vi "TEST VI.vi"() -> ()   [LabVIEW 2010]
uses:
  <vilib>/Utility/miscctls.llb/LVRectTypeDef.ctl
  Visualizer.lvlib
panel:
  in  "OK Button 3":bool
  out "File Data 2":waveform(dbl)[](graph)
  in  "OK Button 2":bool
  out "error out":errorcluster
  in  "OK Button":bool
  out "File Data":waveform(dbl)[](graph)
  in  "File Path":path=path "Q:/VIs/Visualizer/sample.wav"
  in  "Number of Samples/ch":i32=-1
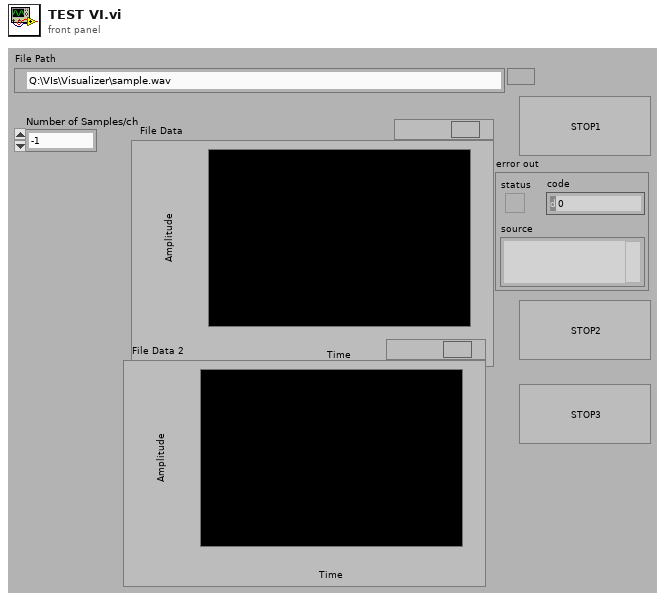
[diagram p1: front panel]
types:
  T1 = typedef "LVRectTypeDef.ctl" = cluster{"Left":i16, "Top":i16, "Right":i16, "Bottom":i16}
  T2 = typedef "Visualizer.lvlib/Visualizer Type ID.ctl" = u32
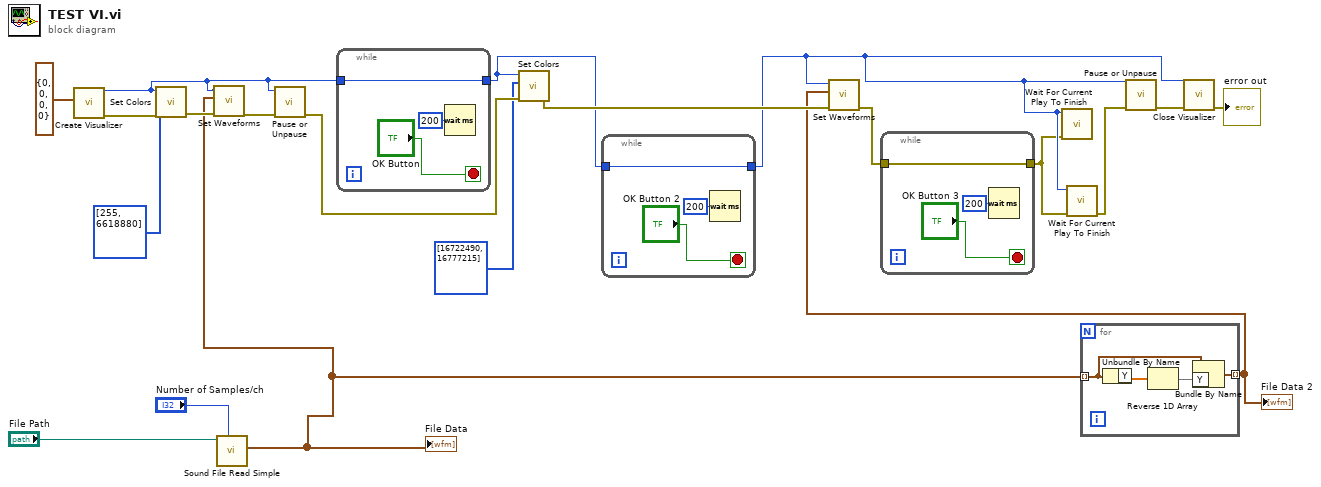
[diagram p0: block diagram]
diagram:
  n1 = call "Create Visualizer.vi"("Front Panel Bounds"=T1 {"Left"=0, "Top"=0, "Right"=0, "Bottom"=0} ("Front Panel Window Bounds")) -> ("error out"=w20:errorcluster, "Visualizer ID"=w14:T2)  [unwired: 9 in]
  n2 = call "Set Colors.vi"("error in (no error)"=w20, "Colors"=u32[] [255, 6618880], "Visualizer ID"=w14) -> ("error out"=w17:errorcluster)  [unwired: 8 in]
  n3 = call <vilib>:"Sound File Read Simple.vi"("number of samples/ch (-1: all)"="Number of Samples/ch", "path"="File Path") -> ("data"=w8:waveform(dbl)[])  [unwired: 6 in, 3 out]
  "File Data" <- w8
  n4 = call "Set Waveforms.vi"("error in (no error)"=w17, "Waveforms"=w8, "Visualizer ID"=w14) -> ("error out"=w15:errorcluster)  [unwired: 8 in]
  n5 = call "Pause or Unpause.vi"("error in (no error)"=w15, "Visualizer ID"=w14) -> ("error out"=w11:errorcluster)  [unwired: 9 in]
  n6 = while {
    tunnel: [w22] -> w6
    tunnel: w14 -> [w22]
    stop <- "OK Button" stop-if-true
    n7 = Wait (ms)(milliseconds to wait=u32 200) -> ()  [unwired: 1 out]
  }
  n8 = call "Set Colors.vi"("error in (no error)"=w11, "Colors"=u32[] [16722490, 16777215], "Visualizer ID"=w6) -> ("error out"=w7:errorcluster)  [unwired: 8 in]
  n9 = while {
    tunnel: [w25] -> w3
    tunnel: w6 -> [w25]
    stop <- "OK Button 2" stop-if-true
    n10 = Wait (ms)(milliseconds to wait=u32 200) -> ()  [unwired: 1 out]
  }
  n11 = for {
    tunnel: w8 -> [w29] mode=indexing
    tunnel: [w27] -> w5 mode=indexing
    n12 = Unbundle By Name(w29) -> ("Y"=w30:dbl[])
    n13 = Reverse 1D Array(array=w30) -> (reversed array=w28:dbl[])
    n14 = Bundle By Name(cluster=w29, "Y"=w28) -> (w27:waveform(dbl))
  }
  "File Data 2" <- w5
  n15 = call "Set Waveforms.vi"("error in (no error)"=w7, "Waveforms"=w5, "Visualizer ID"=w3) -> ("error out"=w4:errorcluster)  [unwired: 8 in]
  n16 = while {
    tunnel: [w32] -> w1
    tunnel: w4 -> [w32]
    stop <- "OK Button 3" stop-if-true
    n17 = Wait (ms)(milliseconds to wait=u32 200) -> ()  [unwired: 1 out]
  }
  n18 = call "Wait For Current Play To Finish.vi"("error in (no error)"=w1, "Visualizer ID"=w3) -> ()  [unwired: 8 in, 2 out]
  n19 = call "Wait For Current Play To Finish.vi"("error in (no error)"=w1, "Visualizer ID"=w3) -> ("error out"=w2:errorcluster)  [unwired: 8 in, 1 out]
  n20 = call "Pause or Unpause.vi"("error in (no error)"=w2, "Visualizer ID"=w3) -> ("error out"=w13:errorcluster)  [unwired: 9 in]
  n21 = call "Close Visualizer.vi"("error in (no error)"=w13, "Visualizer ID"=w3) -> ("error out"=→"error out":errorcluster)  [unwired: 9 in]
